vi "rvc RPY to Rotation Matrix.vi"(9 "type of rotations":u16(ring) items=["Extrinsic", "Intrinsic"], 10 "Convension":u16(ring) items=["XYZ", "ZYX"], 11 "angles":cluster{"roll":dbl, "pitch":dbl, "yaw":dbl}) -> (3 "rotation matrix":T1)   [LabVIEW 2013]
uses:
  <vilib>/Analysis/Matrix/Datatypes/RealMatrix.ctl
  <vilib>/Analysis/coordinate.llb/Euler Rotation Order.ctl
  <vilib>/robotics/Kinematics/NI_Kinematics.lvlib
  <vilib>/Analysis/NI_AALBase.lvlib
  <vilib>/Analysis/baseanly.llb/Real A x B.vi
  <vilib>/Analysis/NI_AALPro.lvlib
  <vilib>/Analysis/Matrix/NI_Matrix.lvlib
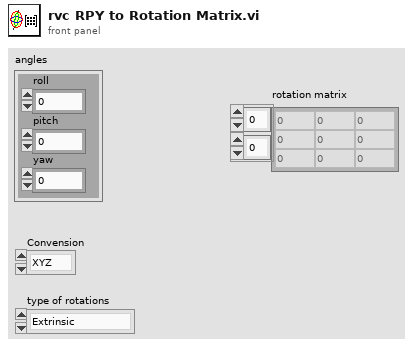
[diagram p1: front panel]
types:
  T1 = typedef "NI_Matrix.lvlib/RealMatrix.ctl" = dbl[][]
  T2 = typedef "NI_AALPro.lvlib/Euler Rotation Order.ctl" = u16
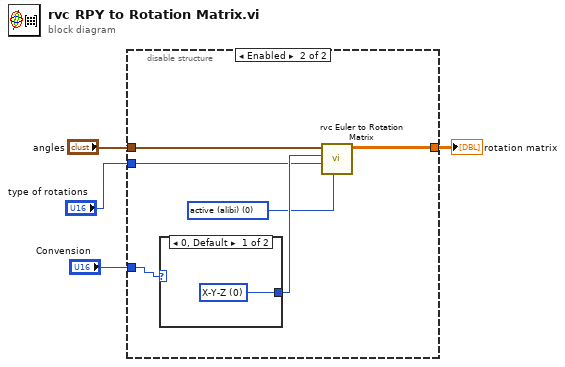
[diagram p0: block diagram]
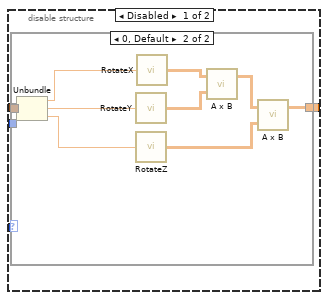
[diagram p2: hidden frame]
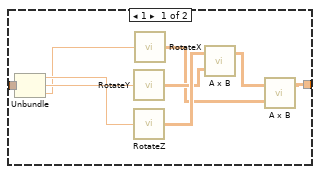
[diagram p3: hidden frame]
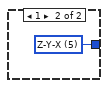
[diagram p4: hidden frame]
diagram:
  n1 = disable-structure shown="Enabled" {
    disable-tunnel: "angles" -> [w7 w31]
    disable-tunnel: [w6 w27] -> w3
    disable-tunnel: "Convension" -> [w5 w30]
    disable-tunnel: "type of rotations" -> [_ w26]
    frame Disabled {
      n2 = case shown="0, Default" w5 {
        tunnel: w7 -> [w16 w25]
        tunnel: [w14 w19] -> w6
        frame 1 {
          n3 = Unbundle(w16) -> ("roll"=w9:dbl, "pitch"=w15:dbl, "yaw"=w8:dbl)
          n4 = call <vilib>:"RotateY.vi"("theta"=w15) -> ("rotation matrix"=w12:T1)
          n5 = call <vilib>:"RotateZ.vi"("theta"=w9) -> ("rotation matrix"=w13:T1)
          n6 = call <vilib>:"RotateX.vi"("theta"=w8) -> ("rotation matrix"=w10:T1)
          n7 = call-poly <vilib>:"A x B.vi"("B"=w12, "A"=w13) -> ("A x B"=w11:T1)  [unwired: 1 out]
          n8 = call-poly <vilib>:"A x B.vi"("B"=w10, "A"=w11) -> ("A x B"=w14:T1)  [unwired: 1 out]
        }
        frame 0, Default {
          n9 = Unbundle(w25) -> ("roll"=w18:dbl, "pitch"=w24:dbl, "yaw"=w17:dbl)
          n10 = call <vilib>:"RotateY.vi"("theta"=w24) -> ("rotation matrix"=w22:T1)
          n11 = call <vilib>:"RotateZ.vi"("theta"=w17) -> ("rotation matrix"=w21:T1)
          n12 = call <vilib>:"RotateX.vi"("theta"=w18) -> ("rotation matrix"=w23:T1)
          n13 = call-poly <vilib>:"A x B.vi"("B"=w22, "A"=w23) -> ("A x B"=w20:T1)  [unwired: 1 out]
          n14 = call-poly <vilib>:"A x B.vi"("B"=w21, "A"=w20) -> ("A x B"=w19:T1)  [unwired: 1 out]
        }
      }
    }
    frame Enabled {
      w28 = u16 0 items=["active (alibi)", "passive (alias)"] ("type of transformation")
      n15 = case shown="0, Default" w30 {
        tunnel: [w32 w33] -> w29
        frame 0, Default {
          w32 = T2 0 items=["X-Y-Z", "X-Z-Y", "Y-X-Z", "Y-Z-X", "Z-X-Y", "Z-Y-X", "X-Y-X", "X-Z-X", "Y-X-Y", "Y-Z-Y", "Z-X-Z", "Z-Y-Z"] ("rotation order")
        }
        frame 1 {
          w33 = T2 5 items=["X-Y-Z", "X-Z-Y", "Y-X-Z", "Y-Z-X", "Z-X-Y", "Z-Y-X", "X-Y-X", "X-Z-X", "Y-X-Y", "Y-Z-Y", "Z-X-Z", "Z-Y-Z"] ("rotation order")
        }
      }
      n16 = call "rvc Euler to Rotation Matrix.vi"("type of transformation"=w28, "type of rotations"=w26, "rotation order"=w29, "euler angles"=w31) -> ("rotation matrix"=w27:T1)  [unwired: 6 in, 1 out]
    }
  }
  "rotation matrix" <- w3
